vi "Sort descending by Version.vi"(11 "Array":string[](array[string])) -> (3 "Sorted Pointers":i32[](array[numeric]))   [LabVIEW 2019]
uses:
  <userlib>/_OpenG.lib/string/string.llb/Trim Whitespace (String Array)__ogtk.vi
  <userlib>/_OpenG.lib/array/array.llb/Filter 1D Array with Scalar (String)__ogtk.vi
  <userlib>/_OpenG.lib/array/array.llb/Sort 1D Array (String)__ogtk.vi
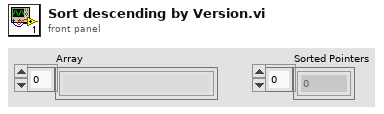
[diagram p1: front panel]
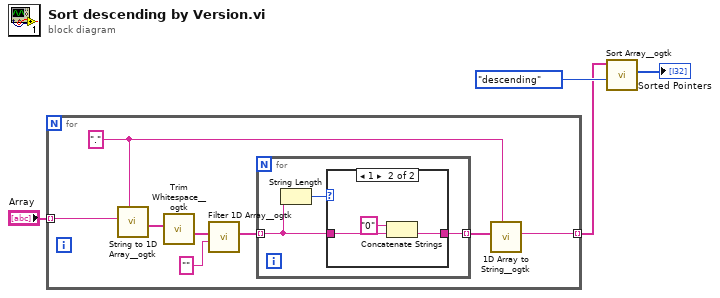
[diagram p0: block diagram]
diagram:
  n1 = for {
    tunnel: [w7] -> w2 mode=indexing
    tunnel: "Array" -> [w5] mode=indexing
    w6 = "." ("delimiter (Tab)")
    n2 = call <userlib>:"String to 1D Array__ogtk.vi"("delimiter (Tab)"=w6, "string"=w5) -> ("Array of Strings"=w12:string[])  [unwired: 9 in]
    n3 = call-poly <userlib>:"Trim Whitespace__ogtk.vi"("String in"=w12) -> ("String out"=w11:string[])  [unwired: 6 in]
    n4 = call-poly <userlib>:"Filter 1D Array__ogtk.vi"("items to filter"="" ("delimiter (Tab)"), "array"=w11) -> ("filtered array"=w9:string[])  [unwired: 4 in, 1 out]
    n5 = for {
      tunnel: w9 -> [w13] mode=indexing
      tunnel: [w14] -> w8 mode=indexing
      n6 = String Length(string=w13) -> (length=w15:i32)
      n7 = case shown="1" w15 {
        tunnel: [w16 w18] -> w14
        tunnel: w13 -> [w16 w19]
        frame Default {
        }
        frame 1 {
          n8 = Concatenate Strings("0" ("string"), w19) -> (w18:string)
        }
      }
    }
    n9 = call <userlib>:"1D Array to String__ogtk.vi"("delimiter (Tab)"=w6, "Array of Strings"=w8) -> ("delimited string"=w7:string)  [unwired: 9 in]
  }
  n10 = call-poly <userlib>:"Sort Array__ogtk.vi"("Order"=enum16{"ascending", "descending"}."descending", "Array in"=w2) -> ("Sorted Pointers"=→"Sorted Pointers":i32[])  [unwired: 8 in, 1 out]
